vi "基础5.vi"() -> ()   [LabVIEW 2014]
panel:
  out "数值":dbl
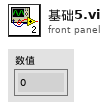
[diagram p1: front panel]
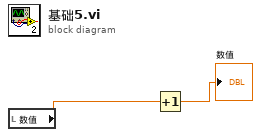
[diagram p0: block diagram]
diagram:
  n1 = local read "数值"() -> (w1:dbl)
  n2 = Increment(x=w1) -> (x+1=→"数值":dbl)
